vi "PI Control (MathScript) cRIO.vi"() -> ()   [LabVIEW 2011]
uses:
  <vilib>/Simulation/Scripting/Companion Diagram/SimConfigNode/SimParams.ctl
  <vilib>/Simulation/Scripting/Companion Diagram/SimConfigNode/_simSolvers.ctl
  <vilib>/Simulation/Implementation/Shared/SIMSCR Execution Mode.ctl
  <vilib>/Platform/TimedLoop/XDataNode/timing_clust.ctl
  <vilib>/Platform/TimedLoop/XDataNode/nitl_modes.ctl
  <vilib>/Platform/TimedLoop/XDataNode/wakeup.ctl
  <vilib>/Simulation/Param Hierarchy/Typedefs/SIMPH Param Control Actions.ctl
  <vilib>/Simulation/Scripting/Editor Utilities/SIM subVI tag data.ctl
  <vilib>/Simulation/Scripting/Editor Utilities/SIM subVI execution type.ctl
  <vilib>/Simulation/Implementation/Shared/NILVSim_FinishedLate.vi
  <vilib>/Simulation/Utility/Implementation/SIM SimulationParams.vi
  <vilib>/Simulation/Nonlinear/Implementation/NILVSim Saturation.llb/SIM Saturation (scalar).vi
  <vilib>/Simulation/Utility/Implementation/SIM Halt.vi
  <vilib>/Simulation/Utility/Implementation/SIM Time.vi
  <vilib>/Simulation/DataSources/Implementation/NILVSim Signal Generator.llb/SIM Signal Generator (scalar).vi
  <vilib>/Simulation/SignalDisplay/Implementation/NILVSim Time Waveform.llb/SIM Time Waveform (vector).vi
  <vilib>/Simulation/ContinuousLinear/Implementation/NILVSim Transfer Function Direct.llb/SIM Transfer Function Direct (SISO CD).vi
  <vilib>/Simulation/Implementation/Shared/SIM Fire Discrete SubVI.vi
  <vilib>/Simulation/Implementation/Shared/NILVSim_Manager.vi
  <vilib>/Simulation/Implementation/Shared/NILVSim_ParamChanged.vi
  <vilib>/Simulation/Implementation/Shared/NILVSim_FinalizeModel.vi
  <vilib>/Simulation/Utility/Implementation/NILVSim SimulationParams (core).vi
  <vilib>/Simulation/Utility/Implementation/NILVSim Get Time and IsAcceptedStep.vi
  <vilib>/Simulation/Implementation/Shared/SIM Fire Discrete SubVI (Core).vi
  <vilib>/imath/engines/lvmath2/RunTimeEngine/ErrorHandling/NIMS_Finalize Error.vi
  <vilib>/imath/engines/lvmath2/RunTimeEngine/RunTimeType/NIMS_RunTimeType_From StrictType (excl LVString).vi
  <instcachedir>/0/NIMS_RunTimeType_From StrictType (excl LVString)_46AE8B54A11948F0BCCEB8091EE7AA4C.lvgen/NIMS_RunTimeType_From StrictType (excl LVString)_46AE8B54A11948F0BCCEB8091EE7AA4C_027.vi
  <vilib>/imath/engines/lvmath2/RunTimeEngine/Struct/NIMS_StructSetField.vi
  <vilib>/imath/engines/lvmath2/RunTimeEngine/Struct/NIMS_StructGetField.vi
  <vilib>/imath/engines/lvmath2/RunTimeEngine/RunTimeType/NIMS_RunTimeType_To Numeric.vi
  <instcachedir>/0/NIMS_RunTimeType_To Numeric_23D8CB4491074484AE5B88877770AD36.lvgen/NIMS_RunTimeType_To Numeric_23D8CB4491074484AE5B88877770AD36_005.vi
  <vilib>/imath/engines/lvmath2/RunTimeEngine/NodeEndStatement/NIMS_NodeEndStatement_Output.vi
  <instcachedir>/0/NIMS_NodeEndStatement_Output_53EC0D466D134D7ABD903AC30B43404B.lvgen/NIMS_NodeEndStatement_Output_53EC0D466D134D7ABD903AC30B43404B_009.vi
  <vilib>/imath/engines/lvmath/Plug In/Control Design/BuiltInFunctions/tf/NIMS_CD_tf(num,den,Ts).vi
  <vilib>/FPGAPlugInAG/cRIO-9113/niLvFpga_Open_cRIO-9113.vi
  <vilib>/Simulation/Implementation/Shared/SIM Unbundle Sim Info.vi
  <vilib>/Simulation/Implementation/Shared/NILVSim_GetModelError.vi
  <vilib>/Simulation/Implementation/Shared/SIM Bundle Sim Info.vi
  <vilib>/Simulation/Implementation/Shared/NILVSim_Initialize.vi
  <vilib>/Utility/error.llb/Error Cluster From Error Code.vi
  <vilib>/rvi/errors/niLvFpgaAdjustHostInterfaceError.vi
  <vilib>/FPGAPlugInAG/cRIO-9113/niLvFpga_Close_cRIO-9113.vi
  <vilib>/Simulation/Scripting/Companion Diagram/SimConfigNode/SimDog.xnode
  <vilib>/addons/Control Design/_Model Construction/Model Typedefs.llb/CD Transfer Function Model (MIMO).ctl
  <vilib>/addons/Control Design/_Model Construction/Model Typedefs.llb/CD General Elements.ctl
  <vilib>/addons/Control Design/_Model Construction/Model Typedefs.llb/CD Transfer Function Model (SISO).ctl
  <vilib>/rvi/interface/nirviOpenFPGA/nirviOpenFPGA.xnode
  <vilib>/Platform/TimedLoop/XDataNode/XDataNode.xnode
  <vilib>/rvi/interface/nirviReadWriteControl/nirviReadWriteControl.xnode
  <vilib>/Simulation/Implementation/XNodeFramework/SimXNode/SimX.xnode
  <vilib>/rvi/interface/nirviCloseFPGA/nirviCloseFPGA.xnode
  NiFpgaLv.dll
  <vilib>/addons/Control Design/_Model Construction/NI_LinSys_Model Typedefs.lvlib
  <vilib>/Platform/TimedLoop/XDataNode/XDNodeRunTimeDep.lvlib
  <vilib>/Simulation/Implementation/Shared/NI_SIM_Implementation.lvlib
panel:
  in  "frequency (Hz)":dbl(slide)=0.4 scale=0.0..10.0
  in  "P":cluster{"Kp":dbl, "Ki":dbl}={"Kp"=5.0, "Ki"=5.0} {"Ki" scale=0.0..15.0; "Kp" scale=0.0..15.0}
  out "Waveform Chart":waveform(dbl)[](graph)
  in  "amplitude (rad)":dbl(slide)=0.52 scale=0.0..3.0
  out "simulation time":dbl=18.68
  in  "stop":bool
  out "Finished Late?":bool
  # "Pulse Train Input"
  # "PI CONTROL GAINS"
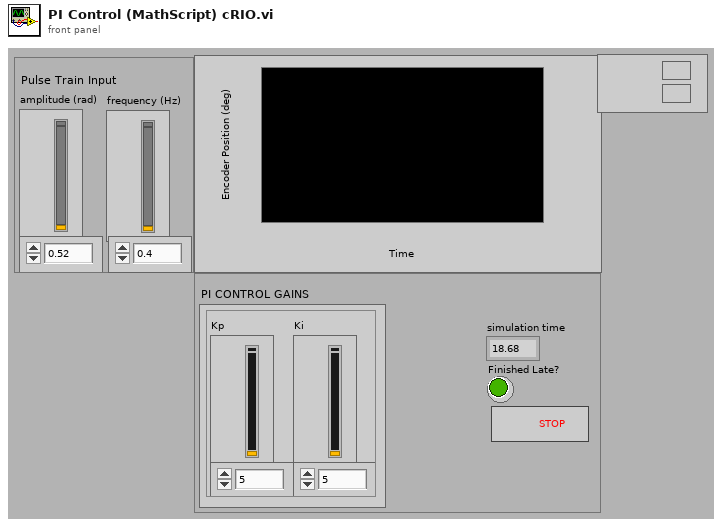
[diagram p1: front panel]
types:
  T1 = typedef "NI_LinSys_Model Typedefs.lvlib/CD Transfer Function Model (MIMO).ctl" = cluster{"properties":T2, "transfer function(s)":T3[][]}
  T2 = typedef "NI_LinSys_Model Typedefs.lvlib/CD General Elements.ctl" = cluster{"Model name":string, "Input names":string[], "Output names":string[], "Input Delays":dbl[], "Output Delays":dbl[], "Sampling Time":dbl, "Notes":string}
  T3 = typedef "NI_LinSys_Model Typedefs.lvlib/CD Transfer Function Model (SISO).ctl" = cluster{"Numerator":dbl[], "Denominator":dbl[], "delay":dbl}
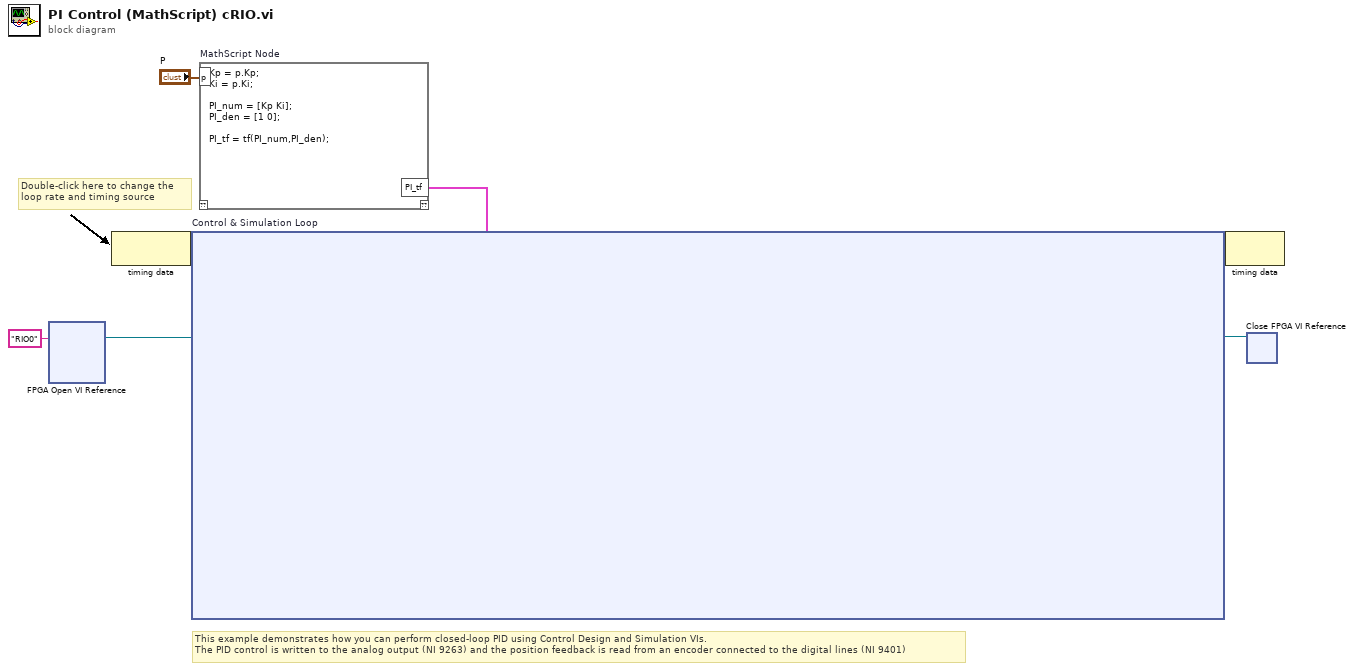
[diagram p0: block diagram]
diagram:
  # "This example demonstrates how you can perform closed-loop PID using Control Design and Simulation VIs.\nThe PID control is written to the analog output (NI 9263) and the position feedback is read from an encoder connected to the digital lines (NI 9401)"
  # "Double-click here to change the\nloop rate and timing source"
  n1 = xnode "FPGA Open VI Reference"("resource name"="RIO0") -> ("FPGA VI Reference Out"=w5:refnum<k20>)  [unwired: 1 in, 1 out]
  n2 = node-c288() -> (w7:variant)  [unwired: 1 in]
  n3 = mathscript code="Kp = p.Kp;\nKi = p.Ki;\n\nPI_num = [Kp Ki];\nPI_den = [1 0];\n\nPI_tf = tf(PI_num,PI_den);"("p"="P") -> ("PI_tf"=w1:T1)  [unwired: 1 in, 1 out]
  n4 = node-c254 "Control & Simulation Loop"(w7, w5, w1) -> (w6:variant, w3:refnum<k20>)
  n5 = node-c288(w6) -> ()  [unwired: 1 out]
  n6 = xnode "Close FPGA VI Reference"("FPGA VI Reference In"=w3) -> ()  [unwired: 1 in, 1 out]
